vi "f_to_c.vi"(1 "Fahrenheit Temperature":dbl) -> (0 "Celsius Temperature":dbl)   [LabVIEW 2023]
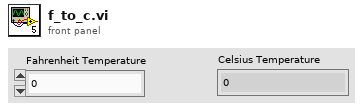
[diagram p1: front panel]
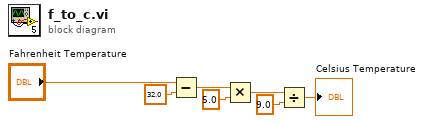
[diagram p0: block diagram]
diagram:
  n1 = Subtract(x="Fahrenheit Temperature", y=32.0 ("x-y")) -> (x-y=w5:dbl)
  n2 = Multiply(x=w5, y=5.0) -> (x*y=w3:dbl)
  n3 = Divide(x=w3, y=9.0) -> (x/y=→"Celsius Temperature":dbl)
